vi "Delete from Array (Multi).vi"(8 "index":i32, 9 "length":i32, 11 "JSON Array In":refnum<class "JSON Array.lvclass">) -> (1 "deleted portion":refnum<class "JSON Datatype.lvclass">[](array[class]), 3 "JSON Array w/ subset deleted":refnum<class "JSON Array.lvclass">)   [LabVIEW 2015, in "LVJSON.lvlib" / "JSON Array.lvclass"]
uses:
  JSON Array.lvclass
  JSON Datatype/JSON Datatype.lvclass
  JSON Array.lvclass/JSON Array.ctl
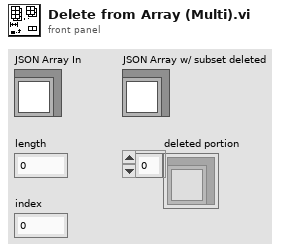
[diagram p1: front panel]
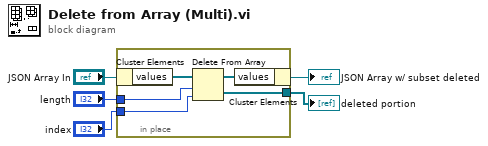
[diagram p0: block diagram]
diagram:
  n1 = in-place {
    in-place-border: "index" -> [w10]
    in-place-border: [w9] -> w1
    in-place-border: "length" -> [w8]
    n2 = in-place-cluster #1("JSON Array In") -> ("values"=w7:refnum<class "JSON Datatype.lvclass">[])
    n3 = Delete From Array(array=w7, length=w8, index=w10) -> (deleted portion=w9:refnum<class "JSON Datatype.lvclass">[], array with subset deleted=w6:refnum<class "JSON Datatype.lvclass">[])
    n4 = in-place-cluster #1("values"=w6) -> (→"JSON Array w/ subset deleted":refnum<class "JSON Array.lvclass">)
  }
  "deleted portion" <- w1
